vi "Register Custom Types.vi"(8 "error in (no error)":errorcluster, 11 "LV-Protoc in":refnum<class "LV-Protoc.lvclass">) -> (0 "error out":errorcluster, 3 "LV-Protoc out":refnum<class "LV-Protoc.lvclass">)   [LabVIEW 2020, in "LV-Protoc.lvlib" / "LV-Protoc.lvclass"]
uses:
  LV-Protoc.lvclass
  LV-Protoc.lvclass/LV-Protoc.ctl
  Custom Type.ctl
  LV-Protoc.lvlib
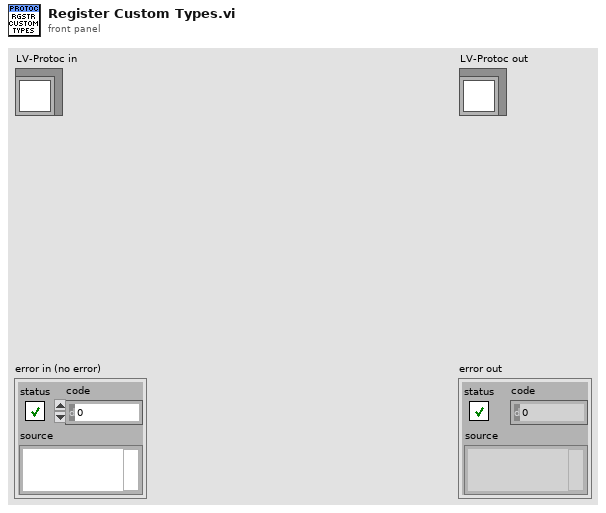
[diagram p1: front panel]
types:
  T1 = typedef "LV-Proto.lvlib/Enumeration.ctl" = cluster{"Name":string, "Values":T2[], "Reserved Numbers":u32[], "Reserved Names":string[]}
  T2 = typedef "LV-Proto.lvlib/Enum Value.ctl" = cluster{"Name":string, "Value":i32}
  T3 = typedef "LV-Proto.lvlib/Message.ctl" = cluster{"Name":string, "Fields":T4[], "Reserved Numbers":u32[], "Reserved Names":string[]}
  T4 = typedef "LV-Proto.lvlib/Field.ctl" = cluster{"Name":string, "Number":u32, "Optional":bool, "Repeated":bool, "Type":T5, "Key Type":T5, "Value Type":T5}
  T5 = typedef "LV-Proto.lvlib/Type.ctl" = cluster{"Type":T6, "Subtype":string}
  T6 = typedef "LV-Proto.lvlib/Proto Type.ctl" = enum16{"UNKNOWN", "double", "float", "int32", "int64", "uint32", "uint64", "sint32", "sint64", "fixed32", "fixed64", "sfixed32", "sfixed64", "bool", "string", "bytes", "enum", "map", "message"}
  T7 = typedef "LV-Protoc.lvlib/Custom Type.ctl" = enum16{"enum", "message"}
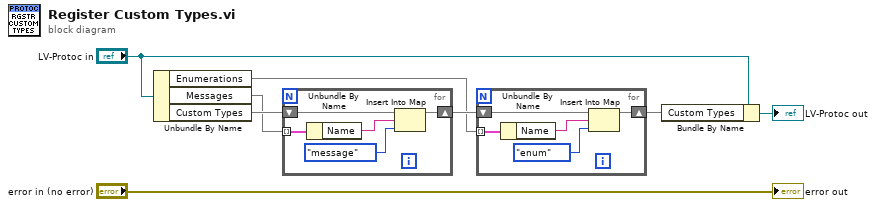
[diagram p0: block diagram]
diagram:
  n1 = Unbundle By Name("LV-Protoc in") -> ("Enumerations"=w5:map{string, T1}, "Messages"=w7:map{string, T3}, "Custom Types"=w8:map{string, T7})
  n2 = for {
    shift-right: [w9] -> w6
    shift-left: w8 -> [w12]
    tunnel: w7 -> [w13] mode=indexing
    n3 = Unbundle By Name(w13) -> ("Name"=w11:string)
    n4 = Insert Into Map(map in=w12, key=w11, value=Custom_Type."message") -> (map out=w9:map{string, T7})  [unwired: 2 out]
  }
  n5 = for {
    shift-right: [w16] -> w3
    shift-left: w6 -> [w18]
    tunnel: w5 -> [w15] mode=indexing
    n6 = Unbundle By Name(w15) -> ("Name"=w14:string)
    n7 = Insert Into Map(map in=w18, key=w14, value=Custom_Type."enum") -> (map out=w16:map{string, T7})  [unwired: 2 out]
  }
  n8 = Bundle By Name(cluster="LV-Protoc in", "Custom Types"=w3) -> (→"LV-Protoc out":refnum<class "LV-Protoc.lvclass">)
  "error out" <- "error in (no error)"
